vi "Get Parameters in Label.vi"(8 "error in":errorcluster, 11 "label ref":T1 format="%.0x") -> (0 "error out":errorcluster, 1 "parameter definitions":T2[](array[typedef]), 2 "parameters":T1[](array[typedef]) format="%.0x", 3 "label ref out":T1 format="%.0x")   [LabVIEW 2024, in "AIM ARINC 429 Scripting.lvlib"]
doc: "Returns all <b>parameters</b> references for the specified <b>label ref</b>."
uses:
  AIM ARINC 429 Scripting.lvlib
  <vilib>/NI VeriStand/Custom Device API/Custom Device Item Ref.ctl
  Shared/Parameter Definition.ctl
  <vilib>/NI/NI VeriStand Encoding and Decoding/Encoding.ctl
  Constants.vi
  <vilib>/NI VeriStand/Custom Device Tools/Custom Device Utility Library/NI VeriStand - Search for Item by GUID.vi
  <vilib>/NI VeriStand/Custom Device Tools/Custom Device Utility Library/Custom Device Utility Library.lvlib
  <vilib>/NI VeriStand/Custom Device API/Custom Device API.lvlib
  <vilib>/NI/NI VeriStand Encoding and Decoding/Encoding and Decoding.lvlib
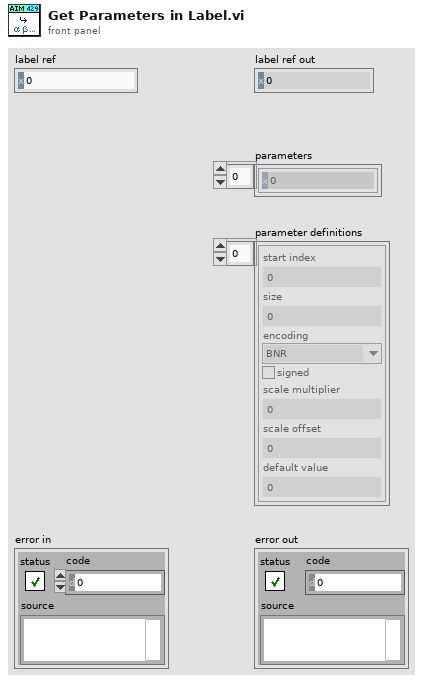
[diagram p1: front panel]
types:
  T1 = typedef "Custom Device API.lvlib/Custom Device Item Ref.ctl" = u64
  T2 = typedef "Parameter Definition.ctl" = cluster{"start index":i32, "size":i32, "encoding":T3, "signed":bool, "scale multiplier":dbl, "scale offset":dbl, "default value":dbl}
  T3 = typedef "Encoding and Decoding.lvlib/Encoding.ctl" = enum16{"BNR", "BCD", "Discrete"}
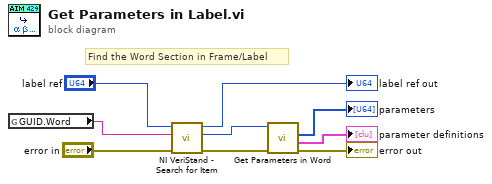
[diagram p0: block diagram]
diagram:
  # "Find the Word Section in Frame/Label"
  n1 = global read "Constants.vi" "GUID.Word"() -> (w3:string)
  n2 = call-poly <vilib>:"NI VeriStand - Search for Item.vi"("error in"="error in", "Item GUID"=w3, "Section Ref in"="label ref") -> ("error out"=w7:errorcluster, "Item Ref"=w6:T1, "Section Ref out"=→"label ref out":T1)  [unwired: 5 in, 1 out]
  n3 = call "Get Parameters in Word.vi"("error in"=w7, "word ref"=w6) -> ("error out"=→"error out":errorcluster, "parameter definitions"=→"parameter definitions":T2[], "parameter refs"=→"parameters":T1[])  [unwired: 6 in, 1 out]
